vi "First.vi"(0 "object in":refnum<class "BFSTreeIterator.lvclass">, 5 "Error In":errorcluster) -> (14 "object out":refnum<class "BFSTreeIterator.lvclass">, 16 "Root":refnum<class "Node.lvclass">, 19 "Error Out":errorcluster)   [LabVIEW 2024, in "BFSTreeIterator.lvclass"]
doc: "Returns root of the collection"
uses:
  BFSTreeIterator.lvclass
  Node_class/Node.lvclass
  BFSTreeIterator.lvclass/BFSTreeIterator.ctl
  Tree_class/Tree.lvclass
panel:
  # "Connector Pane"
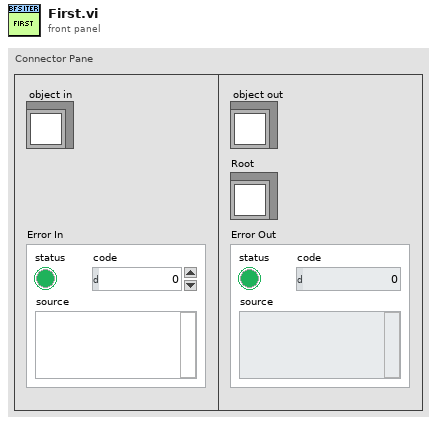
[diagram p1: front panel]
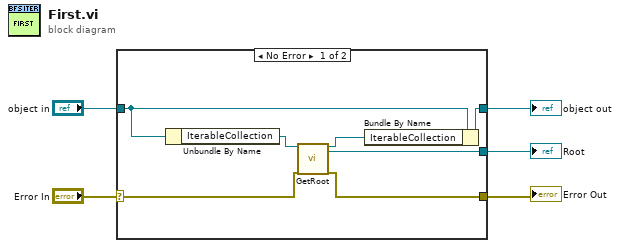
[diagram p0: block diagram]
diagram:
  n1 = case shown="No Error" "Error In" {
    selector: "Error In" -> [w10 w14]
    tunnel: [w9 w14] -> w4
    tunnel: [w7 w13] -> w2
    tunnel: "object in" -> [w12 w13]
    tunnel: [w8 _] -> w1
    frame No Error {
      n2 = Unbundle By Name(w12) -> ("IterableCollection"=w11:refnum<class "Tree.lvclass">)
      n3 = call-dynamic "GetRoot.vi"("object in"=w11, "Error In"=w10) -> ("object out"=w6:refnum<class "Tree.lvclass">, "Root"=w8:refnum<class "Node.lvclass">, "Error Out"=w9:errorcluster)  [unwired: 15 in]
      n4 = Bundle By Name(cluster=w12, "IterableCollection"=w6) -> (w7:refnum<class "BFSTreeIterator.lvclass">)
    }
    frame Error {
    }
  }
  "Error Out" <- w4
  "object out" <- w2
  "Root" <- w1
